vi "Core-DAQ.vi"(7 "Ctrl-Refs":T1, 8 "Err-I":errorcluster, 9 "ErrQRef":refnum<queue>, 11 "DaqQ-I":refnum<queue>) -> (0 "Err-O":errorcluster)   [LabVIEW 2021]
doc: "DAQ LOOP\nMainly handle the hardware I/O."
uses:
  Core-CtrlRefs.ctl
panel:
  # ":: Modularized Parallism Templete ::\n- DAQ LOOP -\nby: Gaoke Yang <gaoke.yang@yahoo.com>\nhttp://www.mViAcademy.com\nCopyright (C) 2010, mVi Academy All Rights Reserved"
  # "Inputs"
  # "Outputs"
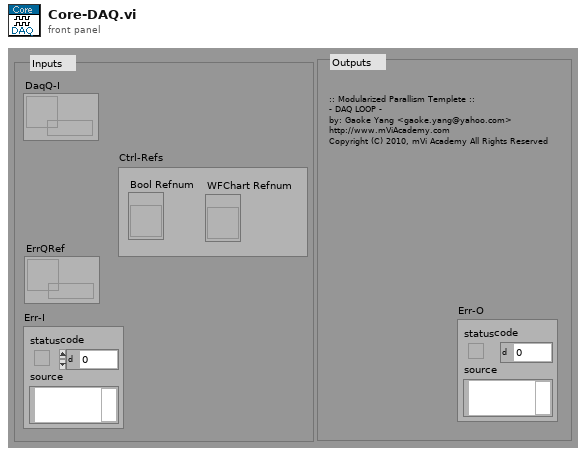
[diagram p1: front panel]
types:
  T1 = typedef "Core-CtrlRefs.ctl" = cluster{"Bool Refnum":refnum<vi>, "WFChart Refnum":refnum<vi>}
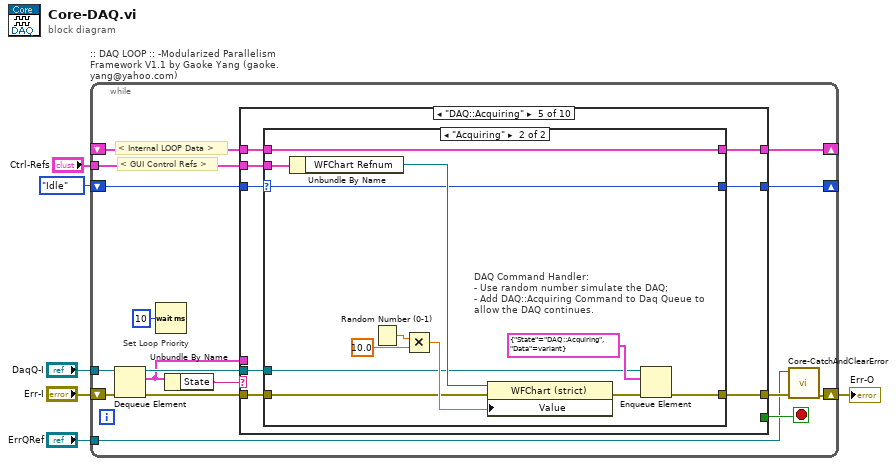
[diagram p0: block diagram]
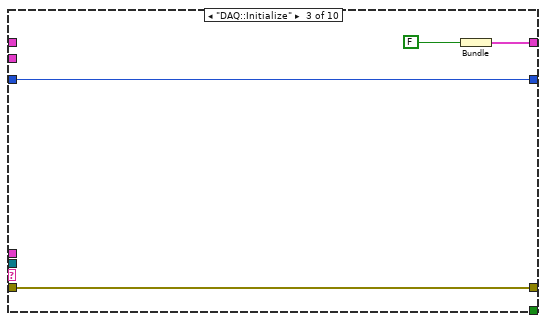
[diagram p4: hidden frame]
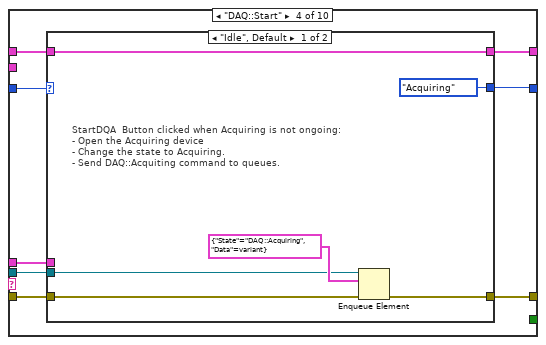
[diagram p5: hidden frame]
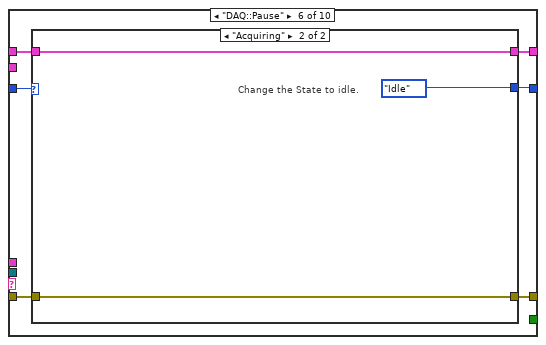
[diagram p8: hidden frame]
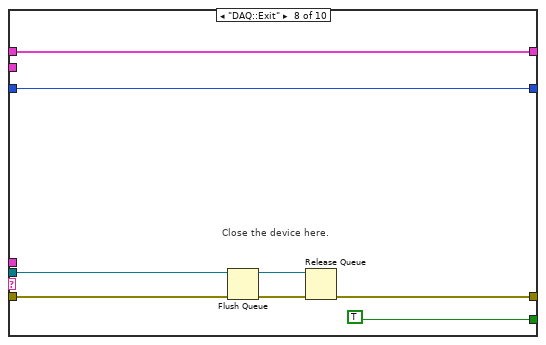
[diagram p11: hidden frame]
diagram:
  n1 = while ":: DAQ LOOP :: -Modularized Parallelism Framework V1.1 by Gaoke Yang (gaoke.yang@yahoo.com)" {
    tunnel: "DaqQ-I" -> [w22]
    shift-right: [w10] -> w3
    shift-left: "Err-I" -> [w17]
    tunnel: "Ctrl-Refs" -> [w15]
    shift-right: [w14] -> _
    shift-left: _ -> [w13]
    tunnel: "ErrQRef" -> [w9]
    shift-right: [w7] -> _
    shift-left: enum16{"Idle", "Acquiring"}."Idle" -> [w8]
    stop <- w20 stop-if-true
    # "Set Loop Priority"
    # "< GUI Control Refs >"
    # "< Internal LOOP Data >"
    n2 = Dequeue Element(queue=w22, error in (no error)=w17) -> (queue out=w19:refnum<queue>, element=w16:cluster{"State":string, "Data":variant}, error out=w21:errorcluster)  [unwired: 2 out]
    n3 = Wait (ms)(milliseconds to wait=u32 10) -> ()  [unwired: 1 out]
    n4 = Unbundle By Name(w16) -> ("State"=w18:string)
    n5 = case shown="\"DAQ::Acquiring\"" w18 {
      tunnel: w21 -> [w24 w28 w30 w35 w56 w77 w86 w94 w98 w101]
      tunnel: [w24 w28 w30 w34 w55 w76 w86 w91 w98 w101] -> w11
      tunnel: [_ _ _ _ _ _ _ TRUE _ _] -> w20
      tunnel: w19 -> [_ _ _ w33 w54 _ _ w93 _ _]
      tunnel: w16 -> [_ _ _ w40 _ _ _ _ _ _]
      tunnel: w15 -> [_ _ _ _ w57 _ _ _ _ _]
      tunnel: [w25 w27 w31 w38 w52 w74 w87 w89 w97 w100] -> w14
      tunnel: w13 -> [w25 w27 _ w39 w53 w75 w87 w89 w97 w100]
      tunnel: w8 -> [w23 w26 w29 w37 w51 w78 w85 w88 w96 w99]
      tunnel: [w23 w26 w29 w36 w50 w73 w85 w88 w96 w99] -> w7
      frame "IDLE", Default {
      }
      frame "-------- DAQ ---------" {
      }
      frame "DAQ::Initialize" {
        n6 = Bundle(FALSE) -> (w31:cluster{bool})  [unwired: 1 in]
      }
      frame "DAQ::Start" {
        n7 = case shown="\"Idle\", Default" w37 {
          selector: w37 -> [_ w48]
          tunnel: [w46 w47] -> w34
          tunnel: w40 -> [_ _]
          tunnel: [w44 w49] -> w38
          tunnel: w39 -> [w44 w49]
          tunnel: [enum16{"Idle", "Acquiring"}."Acquiring" w48] -> w36
          tunnel: w35 -> [w42 w47]
          tunnel: w33 -> [w41 _]
          frame "Idle", Default {
            # "StartDQA  Button clicked when Acquiring is not ongoing:\n- Open the Acquiring device\n- Change the state to Acquiring.\n- Send DAQ::Acquiting command to queues."
            n8 = Enqueue Element(queue=w41, element=cluster{"State":string, "Data":variant} {"State"="DAQ::Acquiring", "Data"=variant} ("DaqQueue"), error in (no error)=w42) -> (error out=w46:errorcluster)  [unwired: 3 out]
          }
          frame "Acquiring" {
            # "The system is already acquiring. \nIgnore the \"Start\" message."
          }
        }
      }
      frame "DAQ::Acquiring" {
        n9 = case shown="\"Acquiring\"" w51 {
          selector: w51 -> [w59 w61]
          tunnel: w57 -> [_ w72]
          tunnel: w56 -> [w58 w66]
          tunnel: [w58 w65] -> w55
          tunnel: w54 -> [_ w64]
          tunnel: w53 -> [w60 w62]
          tunnel: [w60 w62] -> w52
          tunnel: [w59 w61] -> w50
          frame "Idle", Default {
            # "Ignore \"Acquire\" command when the acquisition is idle."
          }
          frame "Acquiring" {
            # "DAQ Command Handler: \n- Use random number simulate the DAQ;\n- Add DAQ::Acquiring Command to Daq Queue to allow the DAQ continues."
            n10 = Unbundle By Name(w72) -> ("WFChart Refnum"=w71:refnum<vi>)
            n11 = Random Number (0-1)() -> (number: 0 to 1=w69:dbl)
            n12 = Multiply(x=w69, y=10.0) -> (x*y=w70:dbl)
            n13 = property class="WFChart (strict)"(reference=w71, error in=w66, "Value"=w70) -> (error out=w63:errorcluster)  [unwired: 1 out]
            n14 = Enqueue Element(queue=w64, element=cluster{"State":string, "Data":variant} {"State"="DAQ::Acquiring", "Data"=variant} ("DaqQueue"), error in (no error)=w63) -> (error out=w65:errorcluster)  [unwired: 3 out]
          }
        }
      }
      frame "DAQ::Pause" {
        n15 = case shown="\"Acquiring\"" w78 {
          selector: w78 -> [w80 _]
          tunnel: [w80 enum16{"Idle", "Acquiring"}."Idle"] -> w73
          tunnel: w75 -> [w81 w83]
          tunnel: [w81 w83] -> w74
          tunnel: w77 -> [w79 w82]
          tunnel: [w79 w82] -> w76
          frame "Idle", Default {
            # "Already idle, ignore Pause command."
          }
          frame "Acquiring" {
            # "Change the State to idle."
          }
        }
      }
      frame "DAQ::UnInitialize" {
      }
      frame "DAQ::Exit" {
        # "Close the device here."
        n16 = Flush Queue(queue=w93, error in (no error)=w94) -> (queue out=w90:refnum<queue>, error out=w92:errorcluster)  [unwired: 1 out]
        n17 = Release Queue(queue=w90, error in (no error)=w92) -> (error out=w91:errorcluster)  [unwired: 1 in, 2 out]
      }
      frame "--------User Case---------" {
      }
      frame "Reserved" {
      }
    }
    n18 = call "Core-CatchAndClearError.vi"("Err-I"=w11, "ErrQ-I"=w9) -> ("Err-O"=w10:errorcluster)  [unwired: 9 in]
  }
  "Err-O" <- w3
